vi "Define_Indexes_Problem_Dots-1.vi"(3 "error IN":errorcluster, 4 "[IN] Index of single track\n(problem displacement)":i32, 5 "[IN] Track\ngroup":T1) -> (0 "error OUT":errorcluster, 1 "[OUT] Index of \nconnected dots\ninside the track":i32[](array[numeric]), 2 "[OUT] Index of connected\ntracks with problem dot":i32[](array[numeric]))   [LabVIEW 2013]
panel:
  in  "[IN]Index of problem\ndisplacement inside track":i32
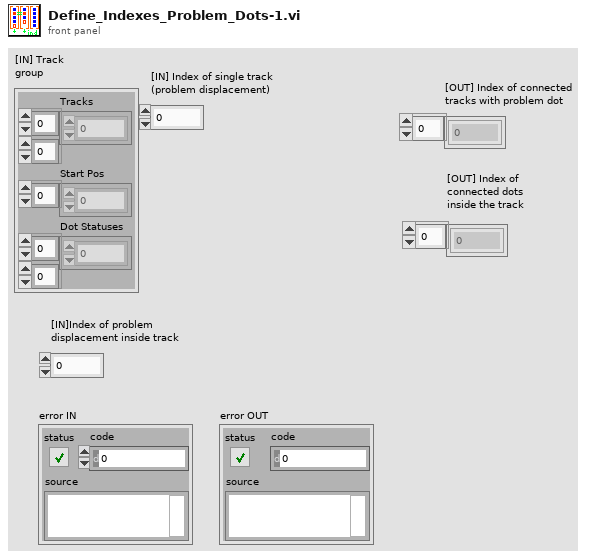
[diagram p1: front panel]
types:
  T1 = cluster{"Tracks":dbl[][], "Start Pos":i32[], "Dot Statuses":i16[][]}
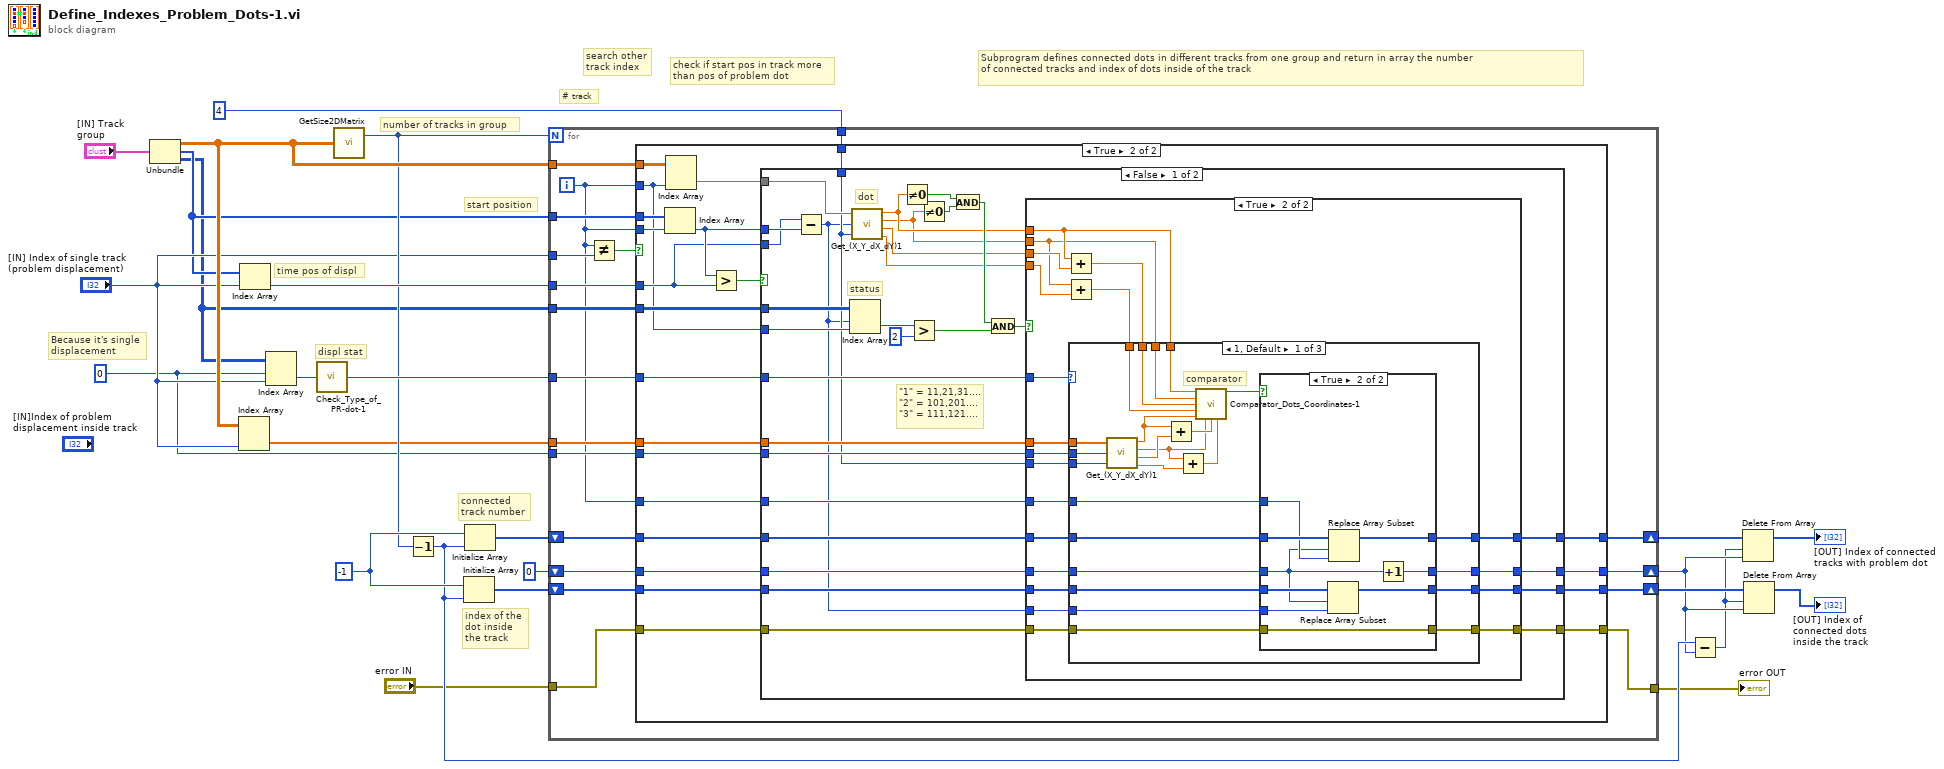
[diagram p0: block diagram]
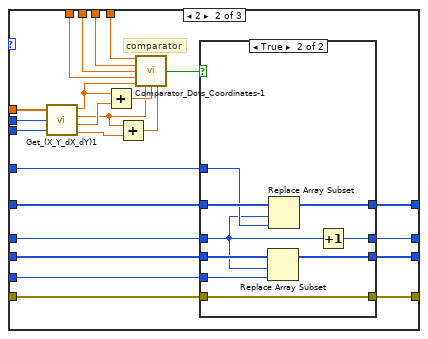
[diagram p5: hidden frame]
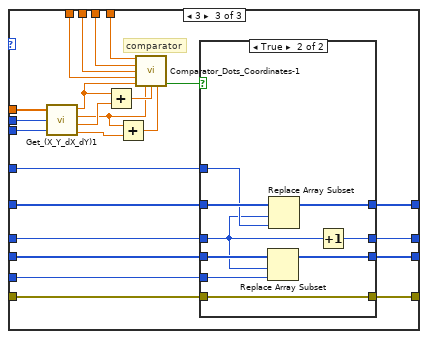
[diagram p7: hidden frame]
diagram:
  w3 = 0 ("index of\ndispl inside\ntrack")
  w20 = -1 ("disabled index (row)")
  # "Because it's single\ndisplacement"
  # "Subprogram defines connected dots in different tracks from one group and return in array the number\nof connected tracks and index of dots inside of the track"
  # "# track"
  # "start position"
  # "number of tracks in group"
  # "check if start pos in track more \nthan pos of problem dot"
  # "search other\ntrack index"
  # "time pos of displ"
  # "index of the dot inside \nthe track"
  # "connected\ntrack number"
  # "displ stat"
  n1 = Unbundle("[IN] Track\ngroup") -> ("Tracks"=w23:dbl[][], "Start Pos"=w14:i32[], "Dot Statuses"=w12:i16[][])
  n2 = Index Array(array=w23, index (col)="[IN] Index of single track\n(problem displacement)") -> (element=w11:dbl[])  [unwired: 1 in]
  n3 = Index Array(array=w14, index="[IN] Index of single track\n(problem displacement)") -> (element=w21:i32)
  n4 = Index Array(array=w12, index (row)=w3, index (col)="[IN] Index of single track\n(problem displacement)") -> (element=w24:i16)
  n5 = call "Check_Type_of_PR-dot-1.vi"("[IN] dot status"=w24) -> ("[OUT] Type of\nproblem dot"=w22:i32)
  n6 = call "GetSize2DMatrix.vi"("Array IN (2D)"=w23) -> ("# Cols"=w19:i32)  [unwired: 1 out]
  n7 = Decrement(x=w19) -> (x-1=w9:i32)
  n8 = Initialize Array(w20, w9) -> (w17:i32[])
  n9 = Initialize Array(w20, w9) -> (w18:i32[])
  n10 = for {
    N: w19 -> [_]
    tunnel: w23 -> [w42]
    tunnel: w22 -> [w38]
    tunnel: w21 -> [w39]
    shift-right: [w30] -> w10
    shift-left: w18 -> [w41]
    shift-right: [w28] -> w8
    shift-left: w17 -> [w40]
    tunnel: "[IN] Index of single track\n(problem displacement)" -> [w44]
    shift-right: [w29] -> w7
    shift-left: 0 -> [w37]
    tunnel: w14 -> [w36]
    tunnel: 4 ("multiplier") -> [w35]
    tunnel: w12 -> [w34]
    tunnel: w11 -> [w33]
    tunnel: w3 -> [w32]
    tunnel: "error IN" -> [w27]
    tunnel: [w26] -> w1
    i -> [w31]
    n11 = Not Equal?(x=w31, y=w44) -> (x != y?=w43:bool)
    n12 = case shown="True" w43 {
      tunnel: w42 -> [_ w70]
      tunnel: w31 -> [_ w61]
      tunnel: w41 -> [w48 w57]
      tunnel: w40 -> [w46 w55]
      tunnel: w39 -> [_ w64]
      tunnel: w38 -> [_ w60]
      tunnel: w37 -> [w47 w56]
      tunnel: w36 -> [_ w69]
      tunnel: w31 -> [_ w68]
      tunnel: w35 -> [_ w63]
      tunnel: w34 -> [_ w62]
      tunnel: w33 -> [_ w59]
      tunnel: w32 -> [_ w58]
      tunnel: w31 -> [_ w54]
      tunnel: [w48 w53] -> w30
      tunnel: [w47 w52] -> w29
      tunnel: [w46 w51] -> w28
      tunnel: w27 -> [w45 w50]
      tunnel: [w45 w49] -> w26
      frame False {
      }
      frame True {
        n13 = Index Array(array=w69, index=w68) -> (element=w65:i32)
        n14 = Index Array(array=w70, index (col)=w61) -> (element=w66:dbl[])  [unwired: 1 in]
        n15 = Greater?(x=w65, y=w64) -> (0:w67:bool)
        n16 = case shown="False" w67 {
          tunnel: w66 -> [w100 _]
          tunnel: w65 -> [w99 _]
          tunnel: w64 -> [w98 _]
          tunnel: w63 -> [w81 _]
          tunnel: w62 -> [w95 _]
          tunnel: w61 -> [w94 _]
          tunnel: w60 -> [w88 _]
          tunnel: w59 -> [w83 _]
          tunnel: w58 -> [w82 _]
          tunnel: w57 -> [w80 w239]
          tunnel: w56 -> [w79 w238]
          tunnel: w55 -> [w78 w237]
          tunnel: w54 -> [w77 _]
          tunnel: [w75 w239] -> w53
          tunnel: [w74 w238] -> w52
          tunnel: [w73 w237] -> w51
          tunnel: w50 -> [w72 w236]
          tunnel: [w71 w236] -> w49
          frame False {
            # "\"1\" = 11,21,31....\n\"2\" = 101,201....\n\"3\" = 111,121...."
            # "status"
            # "dot"
            n17 = Subtract(x=w98, y=w99) -> (x-y=w76:i32)
            n18 = Index Array(array=w95, index (row)=w76, index (col)=w94) -> (element=w93:i16)
            n19 = call "Get_(X_Y_dX_dY)1.vi"("(X,Y,dX,dY)"=w100, "index"=w76, "multiplier"=w81) -> ("X"=w87:dbl, "Y"=w86:dbl, "dX"=w85:dbl, "dY"=w84:dbl)
            n20 = Not Equal To 0?(x=w87) -> (x != 0?=w96:bool)
            n21 = Greater?(x=w93, y=i16 2) -> (0:w90:bool)
            n22 = Not Equal To 0?(x=w86) -> (x != 0?=w97:bool)
            n23 = And(x=w96, y=w97) -> (x .and. y?=w91:bool)
            n24 = And(x=w91, y=w90) -> (x .and. y?=w89:bool)
            n25 = case shown="True" w89 {
              tunnel: w88 -> [_ w124]
              tunnel: w87 -> [_ w118]
              tunnel: w86 -> [_ w117]
              tunnel: w85 -> [_ w120]
              tunnel: w84 -> [_ w119]
              tunnel: w83 -> [_ w123]
              tunnel: w82 -> [_ w122]
              tunnel: w81 -> [_ w121]
              tunnel: w80 -> [w104 w114]
              tunnel: w79 -> [w103 w113]
              tunnel: w78 -> [w102 w112]
              tunnel: w77 -> [_ w111]
              tunnel: w76 -> [_ w110]
              tunnel: [w104 w109] -> w75
              tunnel: [w103 w108] -> w74
              tunnel: [w102 w107] -> w73
              tunnel: w72 -> [w101 w106]
              tunnel: [w101 w105] -> w71
              frame False {
              }
              frame True {
                n26 = Add(x=w118, y=w120) -> (x+y=w116:dbl)
                n27 = Add(x=w117, y=w119) -> (x+y=w115:dbl)
                n28 = case shown="1, Default" w124 {
                  tunnel: w123 -> [w148 w175 w216]
                  tunnel: w122 -> [w147 w174 w215]
                  tunnel: w121 -> [w146 w173 w214]
                  tunnel: w118 -> [w145 w176 w210]
                  tunnel: w117 -> [w144 w177 w211]
                  tunnel: w116 -> [w143 w178 w212]
                  tunnel: w115 -> [w142 w179 w213]
                  tunnel: w114 -> [w134 w170 w208]
                  tunnel: w113 -> [w133 w169 w207]
                  tunnel: w112 -> [w132 w168 w206]
                  tunnel: w111 -> [w131 w171 w209]
                  tunnel: w110 -> [w130 w167 w205]
                  tunnel: [w129 w166 w204] -> w109
                  tunnel: [w128 w165 w203] -> w108
                  tunnel: [w127 w164 w202] -> w107
                  tunnel: w106 -> [w126 w163 w200]
                  tunnel: [w125 w162 w199] -> w105
                  frame 1, Default {
                    # "comparator"
                    n29 = call "Get_(X_Y_dX_dY)1.vi"("(X,Y,dX,dY)"=w148, "index"=w147, "multiplier"=w146) -> ("X"=w141:dbl, "Y"=w138:dbl, "dX"=w140:dbl, "dY"=w137:dbl)
                    n30 = Add(x=w141, y=w140) -> (x+y=w139:dbl)
                    n31 = Add(x=w138, y=w137) -> (x+y=w136:dbl)
                    n32 = call "Comparator_Dots_Coordinates-1.vi"("X1"=w145, "Y1"=w144, "(X+dX)1"=w143, "(Y+dY)1"=w142, "X2"=w141, "Y2"=w138, "(X+dX)2"=w139, "(Y+dY)2"=w136) -> ("X1=X2,Y1=Y2 (1)"=w135:bool)  [unwired: 5 in, 2 out]
                    n33 = case shown="True" w135 {
                      tunnel: w134 -> [w152 w161]
                      tunnel: w133 -> [w151 w157]
                      tunnel: w132 -> [w150 w159]
                      tunnel: w131 -> [_ w160]
                      tunnel: w130 -> [_ w158]
                      tunnel: [w152 w156] -> w129
                      tunnel: [w151 w155] -> w128
                      tunnel: [w150 w154] -> w127
                      tunnel: [w149 w153] -> w125
                      tunnel: w126 -> [w149 w153]
                      frame False {
                      }
                      frame True {
                        n34 = Replace Array Subset(array=w159, new element=w158, index=w157) -> (w154:i32[])
                        n35 = Replace Array Subset(array=w161, new element=w160, index=w157) -> (w156:i32[])
                        n36 = Increment(x=w157) -> (x+1=w155:i32)
                      }
                    }
                  }
                  frame 2 {
                    # "comparator"
                    n37 = call "Get_(X_Y_dX_dY)1.vi"("(X,Y,dX,dY)"=w175, "index"=w174, "multiplier"=w173) -> ("X"=w185:dbl, "Y"=w182:dbl, "dX"=w184:dbl, "dY"=w181:dbl)
                    n38 = Add(x=w185, y=w184) -> (x+y=w183:dbl)
                    n39 = Add(x=w182, y=w181) -> (x+y=w180:dbl)
                    n40 = call "Comparator_Dots_Coordinates-1.vi"("X1"=w176, "Y1"=w177, "(X+dX)1"=w178, "(Y+dY)1"=w179, "X2"=w185, "Y2"=w182, "(X+dX)2"=w183, "(Y+dY)2"=w180) -> ("X1(2)=X2(2),Y1(2)=Y2(2) (2)"=w172:bool)  [unwired: 5 in, 2 out]
                    n41 = case shown="True" w172 {
                      tunnel: w170 -> [w189 w198]
                      tunnel: w169 -> [w188 w194]
                      tunnel: w168 -> [w187 w196]
                      tunnel: w171 -> [_ w197]
                      tunnel: w167 -> [_ w195]
                      tunnel: [w189 w193] -> w166
                      tunnel: [w188 w192] -> w165
                      tunnel: [w187 w191] -> w164
                      tunnel: w163 -> [w186 w190]
                      tunnel: [w186 w190] -> w162
                      frame False {
                      }
                      frame True {
                        n42 = Replace Array Subset(array=w196, new element=w195, index=w194) -> (w191:i32[])
                        n43 = Replace Array Subset(array=w198, new element=w197, index=w194) -> (w193:i32[])
                        n44 = Increment(x=w194) -> (x+1=w192:i32)
                      }
                    }
                  }
                  frame 3 {
                    # "comparator"
                    n45 = call "Get_(X_Y_dX_dY)1.vi"("(X,Y,dX,dY)"=w216, "index"=w215, "multiplier"=w214) -> ("X"=w222:dbl, "Y"=w219:dbl, "dX"=w221:dbl, "dY"=w218:dbl)
                    n46 = Add(x=w222, y=w221) -> (x+y=w220:dbl)
                    n47 = Add(x=w219, y=w218) -> (x+y=w217:dbl)
                    n48 = call "Comparator_Dots_Coordinates-1.vi"("X1"=w210, "Y1"=w211, "(X+dX)1"=w212, "(Y+dY)1"=w213, "X2"=w222, "Y2"=w219, "(X+dX)2"=w220, "(Y+dY)2"=w217) -> ("(1) OR (2) = (3)"=w201:bool)  [unwired: 5 in, 2 out]
                    n49 = case shown="True" w201 {
                      tunnel: w208 -> [w226 w235]
                      tunnel: w207 -> [w225 w231]
                      tunnel: w206 -> [w224 w233]
                      tunnel: w209 -> [_ w234]
                      tunnel: w205 -> [_ w232]
                      tunnel: [w226 w230] -> w204
                      tunnel: [w225 w229] -> w203
                      tunnel: [w224 w228] -> w202
                      tunnel: w200 -> [w223 w227]
                      tunnel: [w223 w227] -> w199
                      frame False {
                      }
                      frame True {
                        n50 = Replace Array Subset(array=w233, new element=w232, index=w231) -> (w228:i32[])
                        n51 = Replace Array Subset(array=w235, new element=w234, index=w231) -> (w230:i32[])
                        n52 = Increment(x=w231) -> (x+1=w229:i32)
                      }
                    }
                  }
                }
              }
            }
          }
          frame True {
          }
        }
      }
    }
  }
  "error OUT" <- w1
  n53 = Subtract(x=w9, y=w7) -> (x-y=w6:i32)
  n54 = Delete From Array(array=w10, length=w6, index=w7) -> (array with subset deleted=→"[OUT] Index of connected\ntracks with problem dot":i32[])  [unwired: 1 out]
  n55 = Delete From Array(array=w8, length=w6, index=w7) -> (array with subset deleted=→"[OUT] Index of \nconnected dots\ninside the track":i32[])  [unwired: 1 out]
